vi "niScope Configure Trigger Digital.vi"(0 "instrument handle":refnum<k15>, 1 "trigger slope":T2 items=["Positive", "Negative"], 5 "trigger source":T1="VAL_RTSI_0", 11 "error in":errorcluster, 12 "trigger holdoff":dbl format="%.4f", 13 "trigger delay":dbl format="%.4f") -> (4 "instrument handle out":refnum<k15>, 15 "error out":errorcluster)   [LabVIEW 2020]
doc: "Configures the common properties of a digital trigger."
uses:
  niScope trigger slope.ctl
  niScope trigger source digital.ctl
  niScope_32.dll
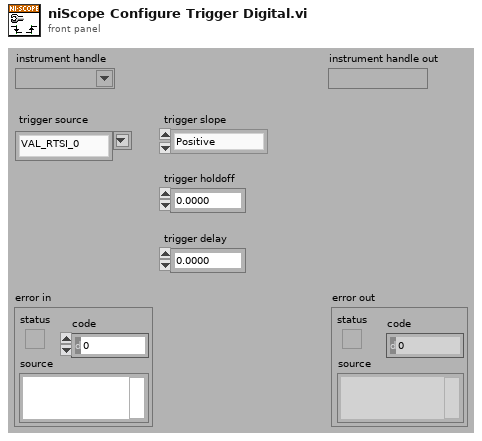
[diagram p1: front panel]
types:
  T1 = typedef "niScope trigger source digital.ctl" = string
  T2 = typedef "niScope trigger slope.ctl" = i32
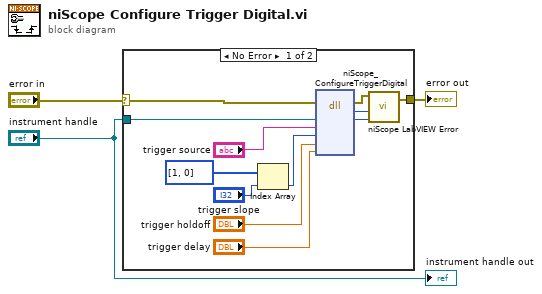
[diagram p0: block diagram]
diagram:
  n1 = case shown="No Error" "error in" {
    selector: "error in" -> [w5 w16]
    tunnel: [w12 w16] -> w3
    tunnel: "instrument handle" -> [w15 _]
    frame No Error {
      n2 = Index Array(array=i32[] [1, 0] ("trigger slope arr"), index="trigger slope") -> (element=w9:i32)
      n3 = dll-call lib="niScope_*.*" fn="niScope_ConfigureTriggerDigital"(error in=w5, "instrument handle"=w15, "triggerSource"="trigger source", "slope"=w9, "holdoff"="trigger holdoff", "delay"="trigger delay") -> (error out=w4:errorcluster, "status"=w14:i32, "instrument handle"=w13:u32)  [unwired: 6 in, 1 out]
      n4 = call "niScope LabVIEW Error.vi"("instrument handle"=w13, "niScope error code (0)"=w14, "error in (no error)"=w4) -> ("error out"=w12:errorcluster)  [unwired: 2 in]
    }
    frame Error {
    }
  }
  "error out" <- w3
  "instrument handle out" <- "instrument handle"
